vi "Turning Point Detection.vi"(6 "Detect Points?":bool, 11 "Input":dbl[](array[numeric])) -> (2 "Points":cluster{i32[], dbl[]}, 3 "Best BSpline Fit":dbl[](array[numeric]))   [LabVIEW 2013, in "main.lvlib"]
uses:
  main.lvlib
  <vilib>/ptbypt/NI_PtbyPt.lvlib
panel:
  out "Residual":dbl
  out "XY Graph":cluster{"Array out":i32[], "Input":dbl[]}[](graph)
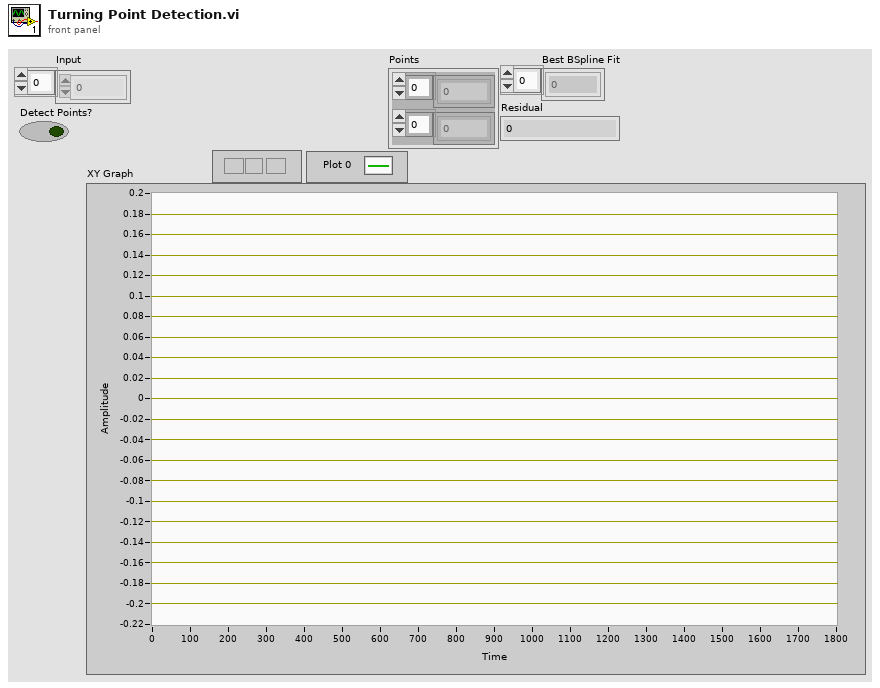
[diagram p1: front panel]
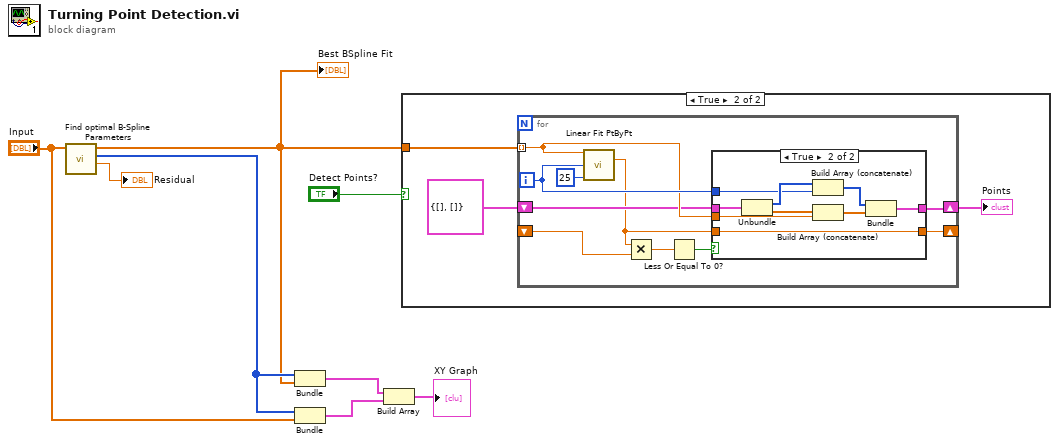
[diagram p0: block diagram]
diagram:
  n1 = call "Find optimal B-Spline Parameters.vi"("Input"="Input") -> ("Residual"=→"Residual":dbl, "X"=w8:i32[], "Best BSpline Fit Y"=w3:dbl[])  [unwired: 8 in]
  "Best BSpline Fit" <- w3
  n2 = Bundle("X"=w8, "Best BSpline Fit Y"=w3) -> (w7:cluster{"X":i32[], "Best BSpline Fit Y":dbl[]})  [unwired: 1 in]
  n3 = Bundle("X"=w8, "Input"="Input") -> (w6:cluster{"X":i32[], "Input":dbl[]})  [unwired: 1 in]
  n4 = Build Array(w7, w6) -> (→"XY Graph":cluster{"X":i32[], "Input":dbl[]}[])
  n5 = case shown="True" "Detect Points?" {
    tunnel: w3 -> [_ w9]
    frame False {
    }
    frame True {
      n6 = for {
        tunnel: w9 -> [w15] mode=indexing
        shift-right: [w18] -> w10
        shift-left: cluster{i32[], dbl[]} {[], []} -> [w14]
        shift-right: [w17] -> _
        shift-left: _ -> [w13]
        i -> [w16]
        n7 = call <vilib>:"Linear Fit PtByPt.vi"("y"=w15, "x"=w16, "sample length"=25) -> ("slope"=w12:dbl)  [unwired: 8 in, 4 out]
        n8 = Multiply(x=w12, y=w13) -> (x*y=w20:dbl)
        n9 = Less Or Equal To 0?(x=w20) -> (x <= 0?=w19:bool)
        n10 = case shown="True" w19 {
          tunnel: [w22 w25] -> w18
          tunnel: w14 -> [w22 w32]
          tunnel: w15 -> [_ w30]
          tunnel: w16 -> [_ w28]
          tunnel: w12 -> [w23 w24]
          tunnel: [w23 w24] -> w17
          frame False {
          }
          frame True {
            n11 = Unbundle(w32) -> (w29:i32[], w31:dbl[])
            n12 = Build Array (concatenate)(w29, w28) -> (w27:i32[])
            n13 = Build Array (concatenate)(w31, w30) -> (w26:dbl[])
            n14 = Bundle(w27, w26) -> (w25:cluster{i32[], dbl[]})  [unwired: 1 in]
          }
        }
      }
      "Points" <- w10
    }
  }
